vi "Send Command.vi"(6 "Timeout (ms)":i32=5000, 8 "error in (no error)":errorcluster, 10 "Data":u64[](array[numeric]) format="%016x", 11 "FPGA Interface in":refnum<class "FPGA Interface.lvclass">) -> (0 "error out":errorcluster)   [LabVIEW 2020, in "BCI-1553 API.lvlib" / "FPGA Interface.lvlib" / "FPGA Interface.lvclass"]
doc: "Sends a pre-formatted command out to a component in the 1553 Session."
uses:
  FPGA Interface.lvclass
  FPGA Interface.lvclass/FPGA Interface.ctl
  <vilib>/Utility/error.llb/Error Cluster From Error Code.vi
  <vilib>/rvi/errors/niLvFpgaAdjustHostInterfaceError.vi
  <vilib>/rvi/interface/nirviMethod/nirviMethod.xnode
  <vilib>/FPGAPlugInAG/Dynamic/niLvFpga_WriteFifo_Dynamic.vi
  <vilib>/rvi/errors/niLvFpgaMergeErrorWithErrorCode.vi
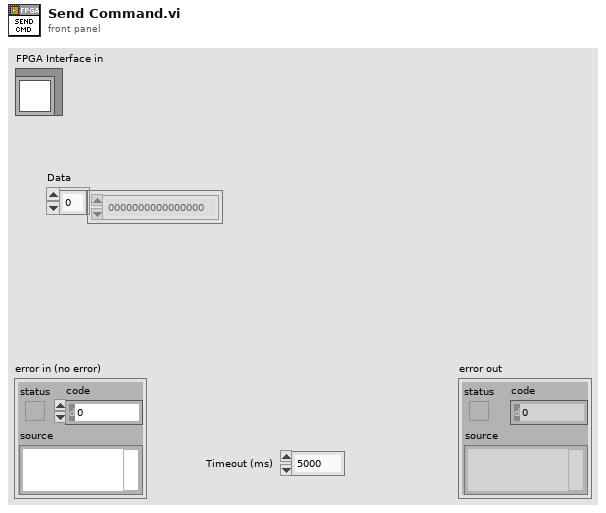
[diagram p1: front panel]
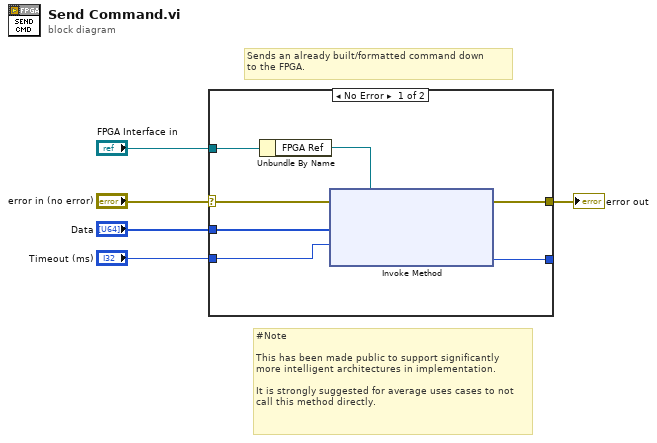
[diagram p0: block diagram]
diagram:
  # "#Note\n\nThis has been made public to support significantly\nmore intelligent architectures in implementation.\n\nIt is strongly suggested for average uses cases to not\ncall this method directly."
  # "Sends an already built/formatted command down\nto the FPGA."
  n1 = case shown="No Error" "error in (no error)" {
    selector: "error in (no error)" -> [w10 w13]
    tunnel: [w9 w13] -> w4
    tunnel: "FPGA Interface in" -> [w12 _]
    tunnel: "Data" -> [w8 _]
    tunnel: "Timeout (ms)" -> [w7 _]
    tunnel: [w6 _] -> _
    frame No Error {
      n2 = Unbundle By Name(w12) -> ("FPGA Ref"=w11:refnum<k20>)
      n3 = xnode "Invoke Method"("FPGA VI Reference In"=w11, "error in"=w10, "Data"=w8, "Timeout (ms)"=w7) -> ("error out"=w9:errorcluster, "Empty Elements Remaining"=w6:u32)  [unwired: 1 out]
    }
    frame Error {
    }
  }
  "error out" <- w4
